vi "Set MPU calib parameters.vi"(6 "Connection Status":T1={"MAC Address"="", "cnx handle"=0, "cnx flags"=0, "Address Type"=125, "Connection Interval (ms)"=125, "Timeout(ms)"=125, "Latency"=0, "bonding handle"=0} {"Address Type" items=["Public", "Random"]}, 7 "Calib file path":path, 8 "Error In":errorcluster, 11 "VISA resource in":refnum<visa-resource-name>) -> (0 "Error Out":errorcluster, 3 "VISA resource out":refnum<visa-resource-name>)   [LabVIEW 2016]
uses:
  <vilib>/BLE/type_def/connection_status_bundle.ctl
  <vilib>/BLE/type_def/address_type.ctl
  Typedef/BLE char handle.ctl
  <vilib>/BLE/ble_functions/ble_write_by_handle_uint8array.vi
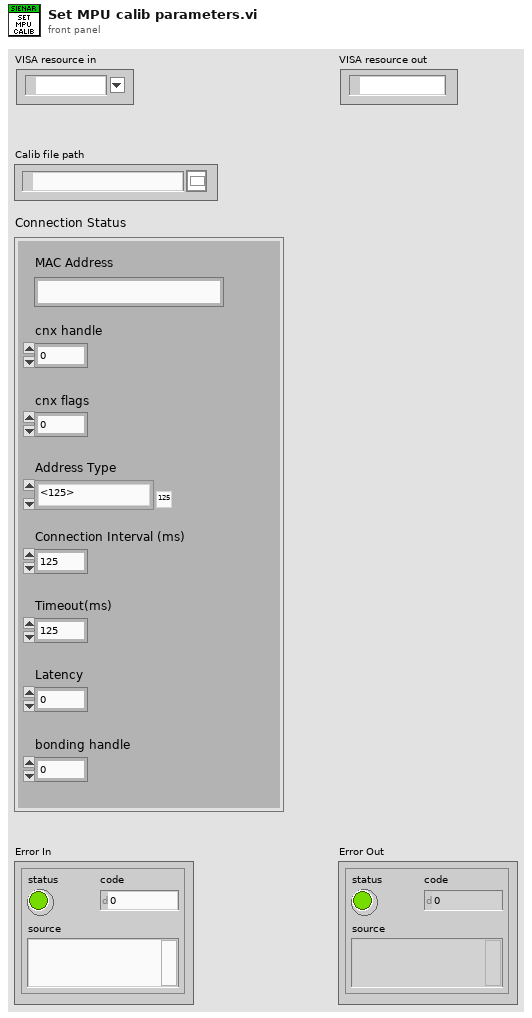
[diagram p1: front panel]
types:
  T1 = typedef "connection_status_bundle.ctl" = cluster{"MAC Address":string, "cnx handle":u8, "cnx flags":u8, "Address Type":T2, "Connection Interval (ms)":u16, "Timeout(ms)":u16, "Latency":u16, "bonding handle":u8}
  T2 = typedef "address_type.ctl" = u8
  T3 = typedef "BLE char handle.ctl" = u16
  T4 = cluster{"Accelerometer":cluster{"Offset":cluster{"X":i16, "Y":i16, "Z":i16}, "Sensitivity":cluster{"X":sgl, "Y":sgl, "Z":sgl}}, "Gyroscope":cluster{"Offset":cluster{"X":i16, "Y":i16, "Z":i16}, "Sensitivity":cluster{"X":sgl, "Y":sgl, "Z":sgl}}, "Magnetometer":cluster{"Offset":cluster{"X":i16, "Y":i16, "Z":i16}, "Sensitivity":cluster{"A11":sgl, "A12":sgl, "A13":sgl, "A22":sgl, "A23":sgl, "A33":sgl}}}
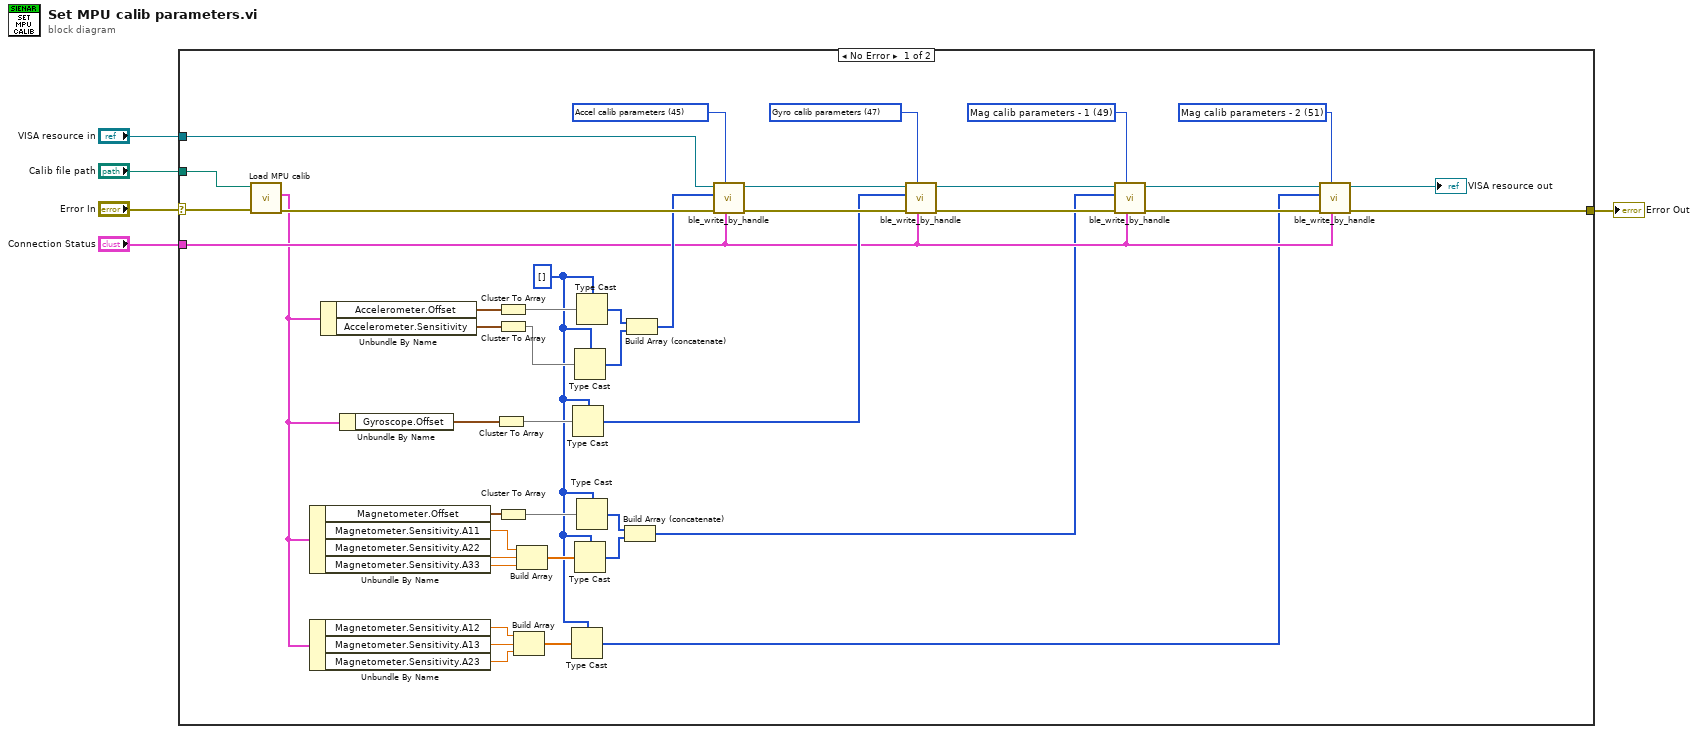
[diagram p0: block diagram]
diagram:
  n1 = case shown="No Error" "Error In" {
    selector: "Error In" -> [w48 w49]
    tunnel: "Calib file path" -> [w47 _]
    tunnel: "VISA resource in" -> [w45 _]
    tunnel: [w24 w49] -> w2
    tunnel: "Connection Status" -> [w26 _]
    frame No Error {
      w6 = T3 51 items=["MPU data"=42, "MPU data - DESCR"=43, "Accel calib parameters"=45, "Gyro calib parameters"=47, "Mag calib parameters - 1"=49, "Mag calib parameters - 2"=51, "YPR"=53, "YPR - DESCR"=54, "Strain sensors"=56, "Strain sensors - DESCR"=57, "Wristband"=59, "Wristband - DESCR"=60] ("BLE char handle")
      w7 = T3 49 items=["MPU data"=42, "MPU data - DESCR"=43, "Accel calib parameters"=45, "Gyro calib parameters"=47, "Mag calib parameters - 1"=49, "Mag calib parameters - 2"=51, "YPR"=53, "YPR - DESCR"=54, "Strain sensors"=56, "Strain sensors - DESCR"=57, "Wristband"=59, "Wristband - DESCR"=60] ("BLE char handle")
      w8 = T3 47 items=["MPU data"=42, "MPU data - DESCR"=43, "Accel calib parameters"=45, "Gyro calib parameters"=47, "Mag calib parameters - 1"=49, "Mag calib parameters - 2"=51, "YPR"=53, "YPR - DESCR"=54, "Strain sensors"=56, "Strain sensors - DESCR"=57, "Wristband"=59, "Wristband - DESCR"=60] ("BLE char handle")
      w9 = T3 45 items=["MPU data"=42, "MPU data - DESCR"=43, "Accel calib parameters"=45, "Gyro calib parameters"=47, "Mag calib parameters - 1"=49, "Mag calib parameters - 2"=51, "YPR"=53, "YPR - DESCR"=54, "Strain sensors"=56, "Strain sensors - DESCR"=57, "Wristband"=59, "Wristband - DESCR"=60] ("BLE char handle")
      w11 = u8[] []
      n2 = call "Load MPU calib.vi"("Error In"=w48, "Calib file path"=w47) -> ("Error Out"=w46:errorcluster, "MPU calib data"=w16:T4)  [unwired: 8 in]
      n3 = Unbundle By Name(w16) -> ("Magnetometer.Offset"=w31:cluster{"X":i16, "Y":i16, "Z":i16}, "Magnetometer.Sensitivity.A11"=w21:sgl, "Magnetometer.Sensitivity.A22"=w22:sgl, "Magnetometer.Sensitivity.A33"=w23:sgl)
      n4 = Unbundle By Name(w16) -> ("Magnetometer.Sensitivity.A12"=w14:sgl, "Magnetometer.Sensitivity.A13"=w15:sgl, "Magnetometer.Sensitivity.A23"=w13:sgl)
      n5 = Unbundle By Name(w16) -> ("Accelerometer.Offset"=w44:cluster{"X":i16, "Y":i16, "Z":i16}, "Accelerometer.Sensitivity"=w43:cluster{"X":sgl, "Y":sgl, "Z":sgl})
      n6 = Unbundle By Name(w16) -> ("Gyroscope.Offset"=w35:cluster{"X":i16, "Y":i16, "Z":i16})
      n7 = Cluster To Array(cluster=w35) -> (array=w34:i16[])
      n8 = Cluster To Array(cluster=w44) -> (array=w42:i16[])
      n9 = Cluster To Array(cluster=w43) -> (array=w41:sgl[])
      n10 = Cluster To Array(cluster=w31) -> (array=w32:i16[])
      n11 = Build Array(w14, w15, w13) -> (w12:sgl[])
      n12 = Build Array(w21, w22, w23) -> (w20:sgl[])
      n13 = Type Cast(type=w11, x=w12) -> (*(type *) &x=w10:u8[])
      n14 = Type Cast(type=w11, x=w34) -> (*(type *) &x=w33:u8[])
      n15 = Type Cast(type=w11, x=w41) -> (*(type *) &x=w39:u8[])
      n16 = Type Cast(type=w11, x=w20) -> (*(type *) &x=w18:u8[])
      n17 = Type Cast(type=w11, x=w42) -> (*(type *) &x=w40:u8[])
      n18 = Type Cast(type=w11, x=w32) -> (*(type *) &x=w19:u8[])
      n19 = Build Array (concatenate)(w19, w18) -> (w17:u8[])
      n20 = Build Array (concatenate)(w40, w39) -> (w38:u8[])
      n21 = call-poly <vilib>:"ble_write_by_handle.vi"("Connection Status"=w26, "Handle"=w9, "error in (no error)"=w46, "data (uint8array)"=w38, "COM Bluegiga in"=w45) -> ("error out"=w37:errorcluster, "COM Bluegiga out"=w36:refnum<visa-resource-name>)  [unwired: 5 in]
      n22 = call-poly <vilib>:"ble_write_by_handle.vi"("Connection Status"=w26, "Handle"=w8, "error in (no error)"=w37, "data (uint8array)"=w33, "COM Bluegiga in"=w36) -> ("error out"=w29:errorcluster, "COM Bluegiga out"=w30:refnum<visa-resource-name>)  [unwired: 5 in]
      n23 = call-poly <vilib>:"ble_write_by_handle.vi"("Connection Status"=w26, "Handle"=w7, "error in (no error)"=w29, "data (uint8array)"=w17, "COM Bluegiga in"=w30) -> ("error out"=w27:errorcluster, "COM Bluegiga out"=w28:refnum<visa-resource-name>)  [unwired: 5 in]
      n24 = call-poly <vilib>:"ble_write_by_handle.vi"("Connection Status"=w26, "Handle"=w6, "error in (no error)"=w27, "data (uint8array)"=w10, "COM Bluegiga in"=w28) -> ("error out"=w24:errorcluster, "COM Bluegiga out"=→"VISA resource out":refnum<visa-resource-name>)  [unwired: 5 in]
    }
    frame Error {
    }
  }
  "Error Out" <- w2
